vi "Prj final.vi"() -> ()   [LabVIEW 2024]
uses:
  <vilib>/DAQmx/read.llb/DAQmx Read (Analog Wfm 1Chan NSamp).vi
  <vilib>/Analysis/baseanly.llb/Mean (DBL).vi
  <vilib>/DAQmx/miscellaneous.llb/DAQmx Fill In Error Info.vi
  <vilib>/measure/macond.llb/FIR Filter for 1 Chan.vi
  <vilib>/Waveform/WDTOps.llb/WDT Get Waveform Subset DBL.vi
  <vilib>/express/express analysis/Spectral/Block/exnSpectralBlock spectral measurements power poly.vi
  <vilib>/express/express analysis/Spectral/Block/exnSpectralBlock spectral measurements power WFM.vi
  <vilib>/express/express analysis/Spectral/XNode/ExpressSpectralMeasurementsBlockNode.xnode
  <vilib>/Analysis/NI_AALBase.lvlib
  <vilib>/measure/NI_MAPro.lvlib
panel:
  out "Waveform used for peak detection":waveform(dbl)(graph)
  in  "Width":i32
  out "Variation BPM":dynamicdata(graph)=[{"t0"=timestamp(3784873284.5436463 s since 1904-01-01), "dt"=0.001, "Y"=array[4400 elements], "attributes"=variant("NI_ChannelName"=variant(string "Tension"), "NI_UnitDescription"=variant(string "Volts"))}, {"t0"=timestamp(3784873284.5436463 s since 1904-01-01), "dt"=0.001, "Y"=array[4400 elements], "attributes"=variant("NI_ChannelName"=variant(string "Tension"), "NI_UnitDescription"=variant(string "Volts"))}, {"t0"=timestamp(3784873284.5436463 s since 1904-01-01), "dt"=0.001, "Y"=array[4400 elements], "attributes"=variant("NI_ChannelName"=variant(string "Tension"), "NI_UnitDescription"=variant(string "Volts"))}]
  out "MOY BPM":dbl
  in  "FIR filter specifications":T1={"Topology"=enum."Off", "Type"=enum."Lowpass", "#Taps"=50, "Lower PB"=100.0, "Upper PB"=0.0, "Lower SB"=200.0, "Upper SB"=0.0} caption="caractéristiques du filtre RIF" {"Lower SB" format="%0.2p"; "Upper SB" format="%0.2p"; "Lower PB" format="%0.2p"; "Upper PB" format="%0.2p"}
  out "F echantillonnage":dbl
  out "Variation Dt":dynamicdata(graph)=[{"t0"=timestamp(3784873284.5436463 s since 1904-01-01), "dt"=0.001, "Y"=array[4400 elements], "attributes"=variant("NI_ChannelName"=variant(string "Tension"), "NI_UnitDescription"=variant(string "Volts"))}, {"t0"=timestamp(3784873284.5436463 s since 1904-01-01), "dt"=0.001, "Y"=array[4400 elements], "attributes"=variant("NI_ChannelName"=variant(string "Tension"), "NI_UnitDescription"=variant(string "Volts"))}, {"t0"=timestamp(3784873284.5436463 s since 1904-01-01), "dt"=0.001, "Y"=array[4400 elements], "attributes"=variant("NI_ChannelName"=variant(string "Tension"), "NI_UnitDescription"=variant(string "Volts"))}]
  in  "Continue":bool
  out "Moy Dt":dbl format="%0.2f"
  out "Input Waveform":waveform(dbl)(graph)
  out "error out":errorcluster caption="sortie d'erreur"
  out "Input Waveform Cutout":waveform(dbl)(graph)
  out "BMP Tone":dbl
  out "Amplitudes Peaks":dbl[](array[numeric])
  out "Temps Peaks":dbl[](array[numeric])
  out "threshold Peaks":dbl format="%0.2f"
  in  "L'aquésition lisible":waveform(dbl)(graph)={"t0"=timestamp(3784873278.9436464 s since 1904-01-01), "dt"=0.001, "Y"=array[10000 elements], "attributes"=variant("NI_ChannelName"=variant(string "Tension"), "NI_UnitDescription"=variant(string "Volts"))}
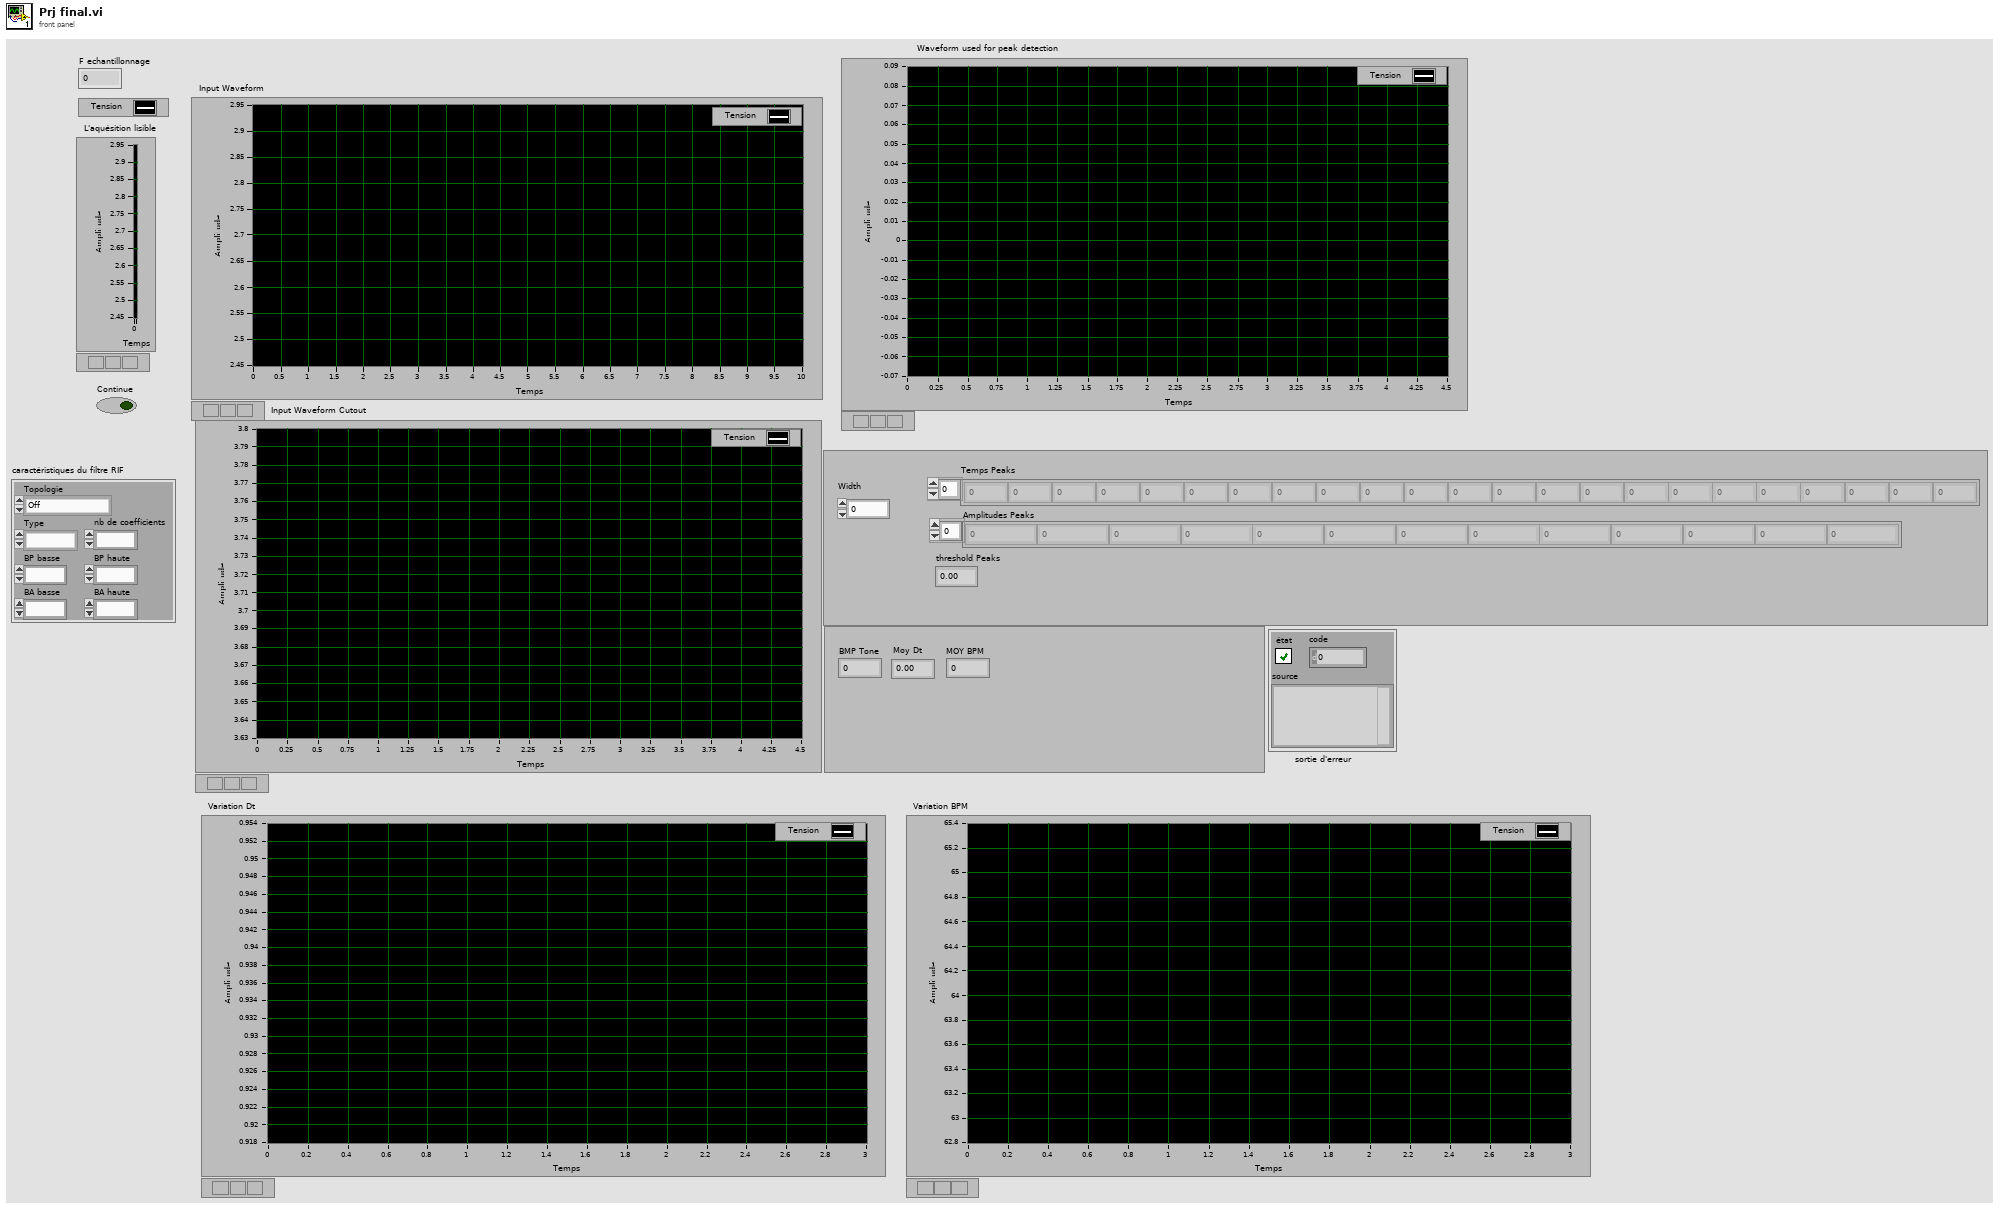
[diagram p1: front panel]
types:
  T1 = cluster{"Topology":enum16{"Off", "FIR by Specification", "Equi-ripple FIR", "Windowed FIR"}, "Type":enum16{"Lowpass", "Highpass", "Bandpass", "Bandstop"}, "#Taps":i32, "Lower PB":dbl, "Upper PB":dbl, "Lower SB":dbl, "Upper SB":dbl}
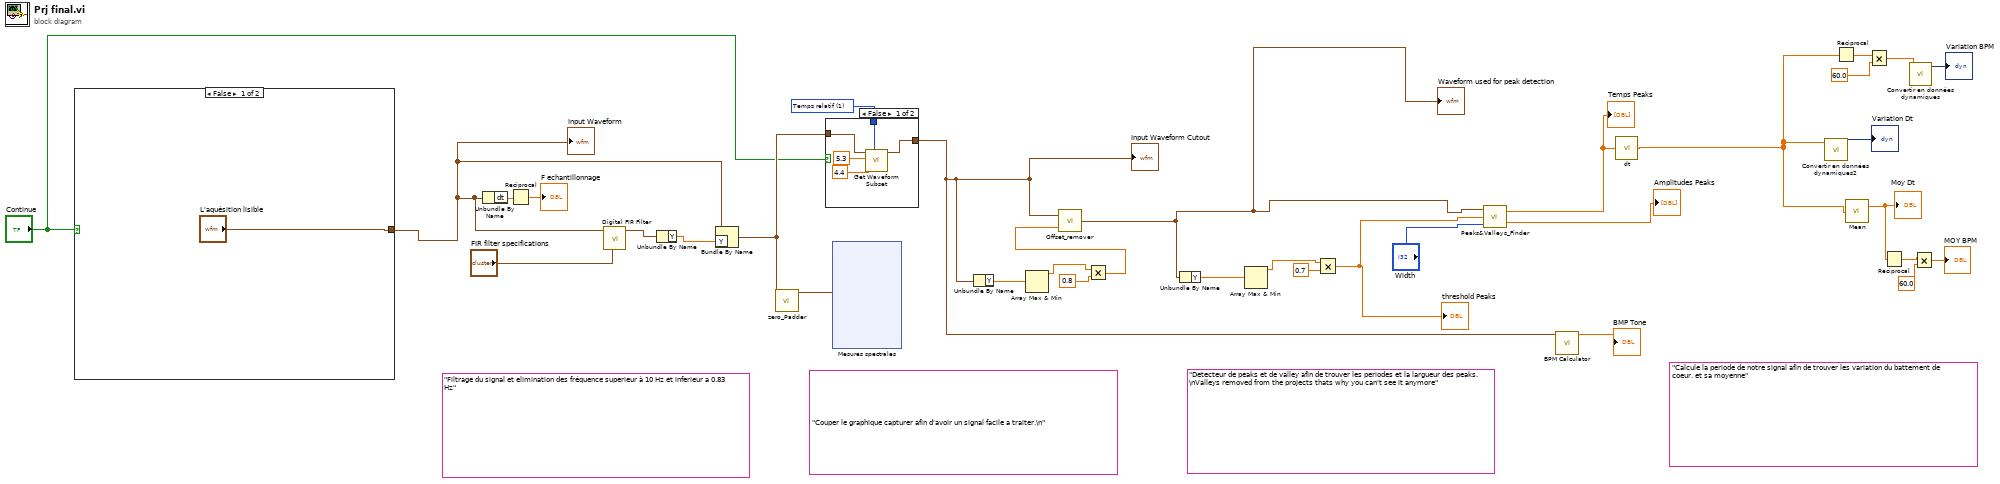
[diagram p0: block diagram]
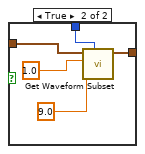
[diagram p2: hidden frame]
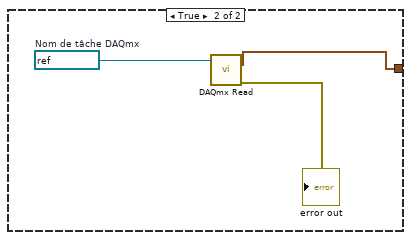
[diagram p3: hidden frame]
diagram:
  (unwired) "Filtrage du signal et elimination des fréquence superieur à 10 Hz et inferieur a 0.83 Hz"
  (unwired) "Detecteur de peaks et de valley afin de trouver les periodes et la largueur des peaks.\nValleys removed from the projects thats why you can't see it anymore"
  (unwired) "Calcule la periode de notre signal afin de trouver les variation du battement de coeur. et sa moyenne"
  (unwired) "Couper le graphique capturer afin d'avoir un signal facile a traiter.\n"
  w15 = u16 1 items=["Échantillons", "Temps relatif"] ("start/duration format")
  n1 = case shown="False" "Continue" {
    tunnel: ["L'aquésition lisible" w36] -> w29
    frame False {
    }
    frame True {
      w38 = refnum<k21> "ECG_IR"  # Nom de tâche DAQmx
      n2 = call-poly <vilib>:"DAQmx Read.vi"("task/channels in"=w38) -> ("data"=w36:waveform(dbl), "error out"=→"error out":errorcluster)  [unwired: 12 in, 1 out]
    }
  }
  "Input Waveform" <- w29
  n3 = Unbundle By Name(w29) -> ("dt"=w31:dbl)
  n4 = Reciprocal(x=w31) -> (1/x=→"F echantillonnage":dbl)
  n5 = call-poly <vilib>:"Digital FIR Filter.vi"("FIR filter specifications"="FIR filter specifications", "signal in"=w29) -> ("signal out"=w26:waveform(dbl))  [unwired: 7 in, 2 out]
  n6 = Unbundle By Name(w26) -> ("Y"=w27:dbl[])
  n7 = Bundle By Name(cluster=w29, "Y"=w27) -> (w25:waveform(dbl))
  n8 = call "zero_Padder.vi"("Graphe en entrée"=w25) -> ("Graphe en sortie"=w34:waveform(dbl))  [unwired: 10 in]
  n9 = case shown="False" "Continue" {
    tunnel: w25 -> [w41 w46]
    tunnel: [w40 w45] -> w8
    tunnel: w15 -> [w39 w44]
    frame False {
      n10 = call-poly <vilib>:"Get Waveform Subset.vi"("start/duration format"=w39, "duration"=4.4, "start samples/time"=5.3, "waveform in"=w41) -> ("waveform out"=w40:waveform(dbl))  [unwired: 2 in, 3 out]
    }
    frame True {
      n11 = call-poly <vilib>:"Get Waveform Subset.vi"("start/duration format"=w44, "duration"=9.0, "start samples/time"=1.0, "waveform in"=w46) -> ("waveform out"=w45:waveform(dbl))  [unwired: 2 in, 3 out]
    }
  }
  "Input Waveform Cutout" <- w8
  n12 = xnode "Mesures spectrales"("Signaux"=w34) -> ()  [unwired: 2 in, 3 out]
  n13 = Unbundle By Name(w8) -> ("Y"=w9:dbl[])
  n14 = Array Max & Min(array=w9) -> (max value=w10:dbl)  [unwired: 3 out]
  n15 = Multiply(x=w10, y=0.8) -> (x*y=w7:dbl)
  n16 = call "Offset_remover.vi"("threshold Peaks"=w7, "Graphe"=w8) -> ("waveform out"=w1:waveform(dbl))
  "Waveform used for peak detection" <- w1
  n17 = Unbundle By Name(w1) -> ("Y"=w12:dbl[])
  n18 = Array Max & Min(array=w12) -> (max value=w13:dbl)  [unwired: 3 out]
  n19 = Multiply(x=w13, y=0.7) -> (x*y=w6:dbl)
  "threshold Peaks" <- w6
  n20 = call "Peaks&Valleys_Finder.vi"("width"="Width", "threshold Peaks"=w6, "waveform in"=w1) -> ("Amplitudes Peaks"=→"Amplitudes Peaks":dbl[], "Locations Peaks"=w2:dbl[])
  "Temps Peaks" <- w2
  n21 = call "BPM Calculator.vi"("waveform in"=w8) -> ("Numeric"=→"BMP Tone":dbl)  [unwired: 10 in]
  n22 = call "dt.vi"("Locations Peaks"=w2) -> ("Tableau"=w3:dbl[])
  n23 = call "Convertir en données dynamiques2"("Array"=w3) -> ("Dynamic Data Type"=→"Variation Dt":dynamicdata)  [unwired: 3 in]
  n24 = Reciprocal(x=w3) -> (1/x=w19:dbl[])
  n25 = call-poly <vilib>:"Mean.vi"("X"=w3) -> ("mean"=w24:dbl)  [unwired: 1 out]
  "Moy Dt" <- w24
  n26 = Multiply(x=w19, y=60.0) -> (x*y=w18:dbl[])
  n27 = Reciprocal(x=w24) -> (1/x=w22:dbl)
  n28 = call "Convertir en données dynamiques"("Array"=w18) -> ("Dynamic Data Type"=→"Variation BPM":dynamicdata)  [unwired: 3 in]
  n29 = Multiply(x=w22, y=60.0) -> (x*y=→"MOY BPM":dbl)
